vi "Insert Channel.vi"(8 "error in (no error)":errorcluster, 9 "ChannelType":T1, 10 "Device Address":tag, 11 "Sequencer in":refnum<class "Sequencer.lvclass">) -> (0 "error out":errorcluster, 3 "Sequencer out":refnum<class "Sequencer.lvclass">)   [LabVIEW 2015, in "Sequencer.lvlib" / "Sequencer.lvclass"]
uses:
  Sequencer.lvclass
  <vilib>/ActorFramework/Actor/Actor.lvclass
  Channel/ChannelInfo.lvclass
  Channel/ChannelConfig.lvclass
  Channel/Channel/Channel.lvclass
  <vilib>/ErrorRing/Error Ring.xnode
  <vilib>/Utility/error.llb/Error Cluster From Error Code.vi
  SequencerConfig.lvclass
  SequencerInfo.lvclass
  ChannelTypes.ctl
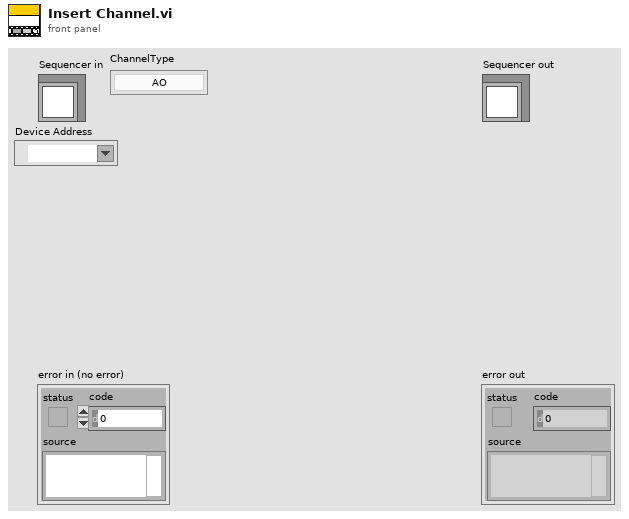
[diagram p1: front panel]
types:
  T1 = typedef "Sequencer.lvlib/Sequencer.lvclass/ChannelTypes.ctl" = enum16{"AO", "DO", "AI"}
  T2 = cluster{"Accessors:Sample Rate":dbl, "Accessors:Buffer Size":dbl}
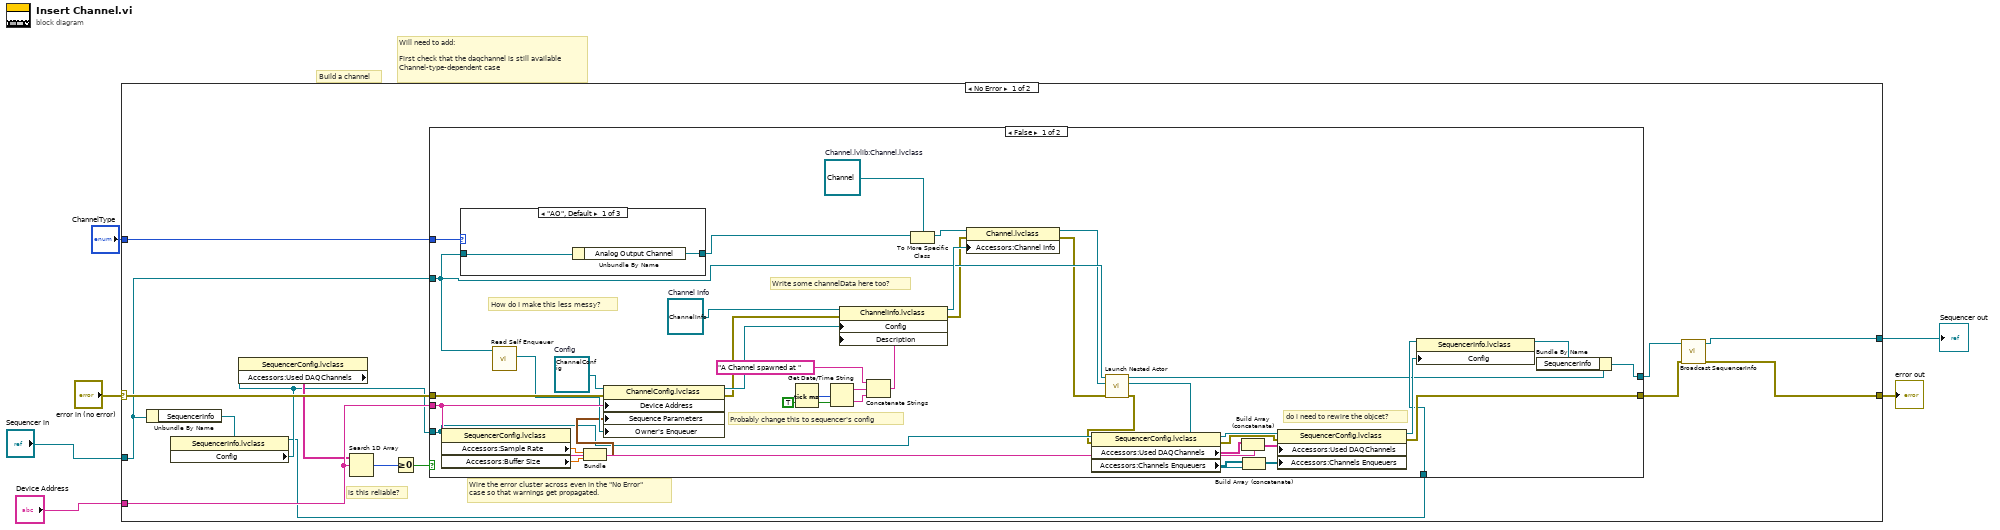
[diagram p0: block diagram]
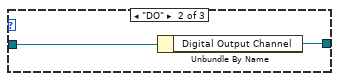
[diagram p2: hidden frame]
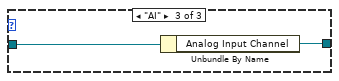
[diagram p3: hidden frame]
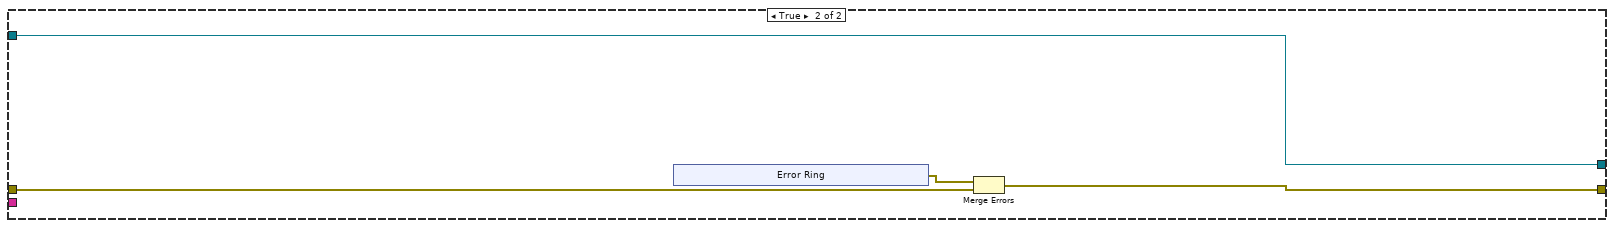
[diagram p4: hidden frame]
diagram:
  # "Will need to add:\n\nFirst check that the daqchannel is still available\nChannel-type-dependent case"
  # "Build a channel"
  n1 = case shown="No Error" "error in (no error)" {
    selector: "error in (no error)" -> [w20 w77]
    tunnel: [w11 w77] -> w5
    tunnel: [w13 w76] -> w3
    tunnel: "Sequencer in" -> [w18 w76]
    tunnel: "Device Address" -> [w17 _]
    tunnel: "ChannelType" -> [w19 _]
    frame No Error {
      # "is this reliable?"
      # "Wire the error cluster across even in the \"No Error\"\ncase so that warnings get propagated."
      n2 = Unbundle By Name(w18) -> ("SequencerInfo"=w10:refnum<class "SequencerInfo.lvclass">)
      n3 = property class="SequencerInfo.lvclass"(reference=w10) -> (reference out=w7:refnum<class "SequencerInfo.lvclass">, "Config"=w8:refnum<class "SequencerConfig.lvclass">)  [unwired: 1 in, 1 out]
      n4 = property class="SequencerConfig.lvclass"(reference=w8) -> ("Accessors:Used DAQChannels"=w9:tag[])  [unwired: 1 in, 2 out]
      n5 = Search 1D Array(1D array=w9, element=w17) -> (index of element=w16:i32)  [unwired: 1 in]
      n6 = Greater Or Equal To 0?(x=w16) -> (x >= 0?=w15:bool)
      n7 = case shown="False" w15 {
        tunnel: w20 -> [w49 w67]
        tunnel: [w25 w70] -> w14
        tunnel: [w30 w68] -> w12
        tunnel: w19 -> [w55 _]
        tunnel: w18 -> [w53 w70]
        tunnel: w17 -> [w52 _]
        tunnel: w8 -> [w37 _]
        tunnel: w7 -> [w27 _]
        frame False {
          w56 = refnum<class "Channel.lvclass"> refnum  # Channel.lvlib:Channel.lvclass
          w57 = refnum<class "ChannelConfig.lvclass"> refnum  # Config
          w60 = refnum<class "ChannelInfo.lvclass"> refnum  # Channel Info
          # "How do I make this less messy?"
          # "Write some channelData here too?"
          # "do i need to rewire the objcet?"
          # "Probably change this to sequencer's config"
          n8 = property class="SequencerConfig.lvclass"(reference=w37) -> ("Accessors:Sample Rate"=w40:dbl, "Accessors:Buffer Size"=w39:dbl)  [unwired: 1 in, 2 out]
          n9 = case shown="\"AO\", Default" w55 {
            tunnel: [w62 w63 w66] -> w54
            tunnel: w53 -> [w61 w64 w65]
            frame "AO", Default {
              n10 = Unbundle By Name(w61) -> ("Analog Output Channel"=w62:refnum<class "Analog Output Channel.lvclass">)
            }
            frame "DO" {
              n11 = Unbundle By Name(w64) -> ("Digital Output Channel"=w63:refnum<class "Digital Output Channel.lvclass">)
            }
            frame "AI" {
              n12 = Unbundle By Name(w65) -> ("Analog Input Channel"=w66:refnum<class "Analog Input Channel.lvclass">)
            }
          }
          n13 = call <vilib>:"Read Self Enqueuer.vi"("Actor"=w53) -> ("Self Enqueuer"=w46:refnum<class "Message Enqueuer.lvclass">)  [unwired: 10 in]
          n14 = Bundle("Accessors:Sample Rate"=w40, "Accessors:Buffer Size"=w39) -> (w38:T2)  [unwired: 1 in]
          n15 = property class="ChannelConfig.lvclass"(reference=w57, error in=w49, "Device Address"=w52, "Sequence Parameters"=w38, "Owner's Enqueuer"=w46) -> (reference out=w58:refnum<class "ChannelConfig.lvclass">, error out=w51:errorcluster)
          n16 = Tick Count (ms)() -> (millisecond timer value=w45:u32)
          n17 = Get Date/Time String(seconds (now)=w45, want seconds? (F)=TRUE) -> (date string=w44:string, time string=w43:string)  [unwired: 1 in]
          n18 = Concatenate Strings("A Channel spawned at " ("Description"), w44, w43) -> (w41:string)
          n19 = property class="ChannelInfo.lvclass"(reference=w60, error in=w51, "Config"=w58, "Description"=w41) -> (reference out=w59:refnum<class "ChannelInfo.lvclass">, error out=w50:errorcluster)
          n20 = To More Specific Class(target class=w56, reference=w54) -> (specific class reference=w23:refnum<class "Channel.lvclass">)  [unwired: 1 in, 1 out]
          n21 = property class="Channel.lvclass"(reference=w23, error in=w50, "Accessors:Channel Info"=w59) -> (reference out=w22:refnum<class "Channel.lvclass">, error out=w48:errorcluster)
          n22 = call <vilib>:"Launch Nested Actor.vi"("error in (no error)"=w48, "Nested Actor"=w22, "Caller Actor in"=w53) -> ("error out"=w29:errorcluster, "Nested Actor's Enqueuer"=w47:refnum<class "Message Enqueuer.lvclass">, "Caller Actor out"=w26:refnum<class "Sequencer.lvclass">)  [unwired: 6 in]
          n23 = property class="SequencerConfig.lvclass"(reference=w37, error in=w29) -> (reference out=w32:refnum<class "SequencerConfig.lvclass">, error out=w31:errorcluster, "Accessors:Used DAQChannels"=w35:tag[], "Accessors:Channels Enqueuers"=w36:refnum<class "Message Enqueuer.lvclass">[])
          n24 = Build Array (concatenate)(w35, w52) -> (w34:tag[])
          n25 = Build Array (concatenate)(w36, w47) -> (w33:refnum<class "Message Enqueuer.lvclass">[])
          n26 = property class="SequencerConfig.lvclass"(reference=w32, error in=w31, "Accessors:Used DAQChannels"=w34, "Accessors:Channels Enqueuers"=w33) -> (reference out=w28:refnum<class "SequencerConfig.lvclass">, error out=w30:errorcluster)
          n27 = property class="SequencerInfo.lvclass"(reference=w27, "Config"=w28) -> (reference out=w24:refnum<class "SequencerInfo.lvclass">)  [unwired: 1 in, 1 out]
          n28 = Bundle By Name(cluster=w26, "SequencerInfo"=w24) -> (w25:refnum<class "Sequencer.lvclass">)
        }
        frame True {
          n29 = xnode "Error Ring"() -> ("error out"=w69:errorcluster)
          n30 = Merge Errors(w69, w67) -> (w68:errorcluster)
        }
      }
      n31 = call "Broadcast SequencerInfo.vi"("error in (no error)"=w12, "Sequencer in"=w14) -> ("error out"=w11:errorcluster, "Sequencer out"=w13:refnum<class "Sequencer.lvclass">)  [unwired: 8 in]
    }
    frame Error {
    }
  }
  "error out" <- w5
  "Sequencer out" <- w3
